vi "DAC Save Results.vi"(8 "error in":errorcluster, 9 "Log Details?":bool, 10 "tdms file":refnum<k34>, 11 "DAC TEG Temp in":refnum<class "DAC TEG Temp.lvclass">) -> (0 "error out":errorcluster)   [LabVIEW 2019, in "DAC.lvlib" / "DAC TEG Temp.lvclass"]
uses:
  DAC TEG Temp.lvclass
  C:/Users/krio/Documents/LV_Projects/test-stand/App/DAC/DAC.lvclass
  DAC.lvclass/DAC.ctl
  DAC TEG Temp.lvclass/DAC TEG Temp.ctl
  DAC.lvclass
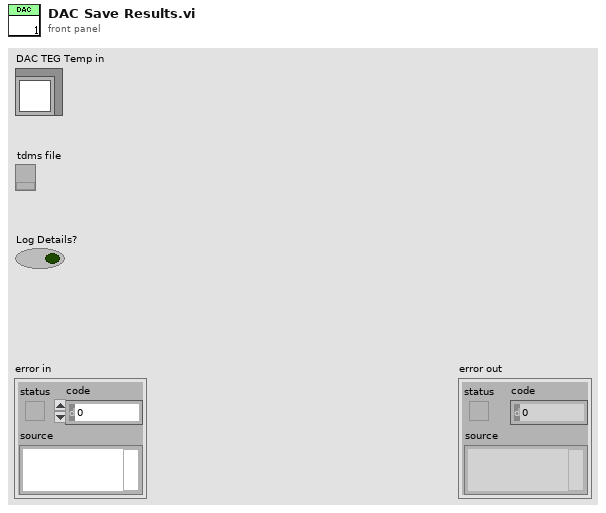
[diagram p1: front panel]
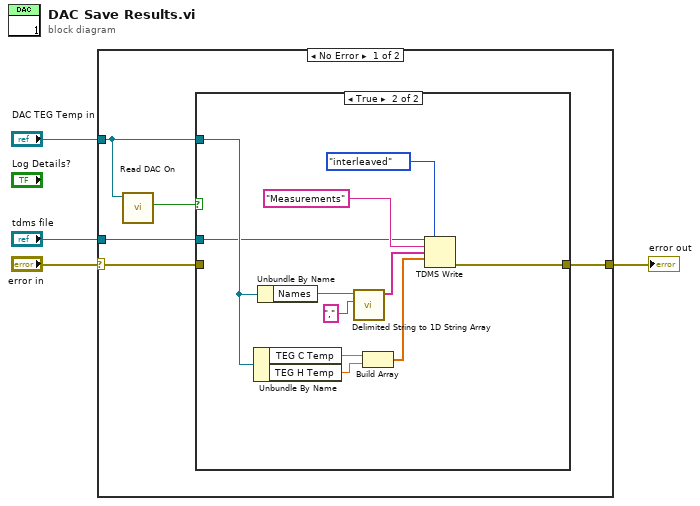
[diagram p0: block diagram]
diagram:
  n1 = case shown="No Error" "error in" {
    selector: "error in" -> [w6 w22]
    tunnel: "DAC TEG Temp in" -> [w9 _]
    tunnel: "tdms file" -> [w7 _]
    tunnel: [w5 w22] -> w1
    frame No Error {
      n2 = call "Read DAC On.vi"("DAC in"=w9) -> ("DAC On"=w8:bool)  [unwired: 8 in, 2 out]
      n3 = case shown="True" w8 {
        tunnel: w9 -> [_ w14]
        tunnel: w7 -> [_ w12]
        tunnel: w6 -> [w10 _]
        tunnel: [w10 w15] -> w5
        frame False {
        }
        frame True {
          n4 = Unbundle By Name(w14) -> ("TEG C Temp"=w18:dbl, "TEG H Temp"=w17:dbl)
          n5 = Unbundle By Name(w14) -> ("Names"=w20:string)
          n6 = call <vilib>:"Delimited String to 1D String Array.vi"("delimiter"=",", "delimited string"=w20) -> ("string array"=w19:string[])  [unwired: 9 in]
          n7 = Build Array(w18, w17) -> (w16:dbl[])
          n8 = TDMS Write(0:w12, 1:enum16{"decimated", "interleaved"}."interleaved" ("data layout (0:decimated)"), 5:"Measurements" ("group name in (Untitled)"), 7:w19, 9:w16) -> (15:w15:errorcluster)  [unwired: 1 in, 3 out]
        }
      }
    }
    frame Error {
    }
  }
  "error out" <- w1
